vi "init.vi"(10 "Size":u32, 11 "Key Value Pairs":T1[](array[typedef])) -> (0 "error out":errorcluster, 3 "Bucket out":refnum<class "Bucket.lvclass">)   [LabVIEW 2017, in "Bucket.lvclass"]
uses:
  <userlib>/836-Library/Data_Structures/Bucket/Bucket.lvclass
  <userlib>/836-Library/Data_Structures/Bucket/Types/KeyValuePair.ctl
  <userlib>/836-Library/Data_Structures/Bucket/Bucket.lvclass/Bucket.ctl
  <vilib>/Utility/error.llb/Error Cluster From Error Code.vi
  <vilib>/ErrorRing/Error Ring.xnode
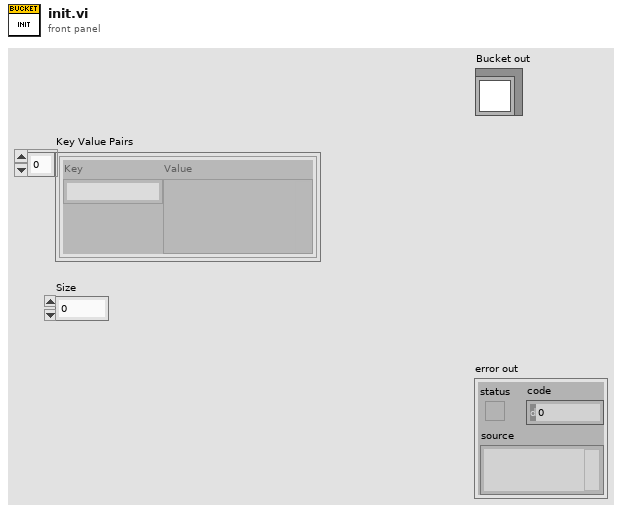
[diagram p1: front panel]
types:
  T1 = typedef "KeyValuePair.ctl" = cluster{"Key":string, "Value":variant}
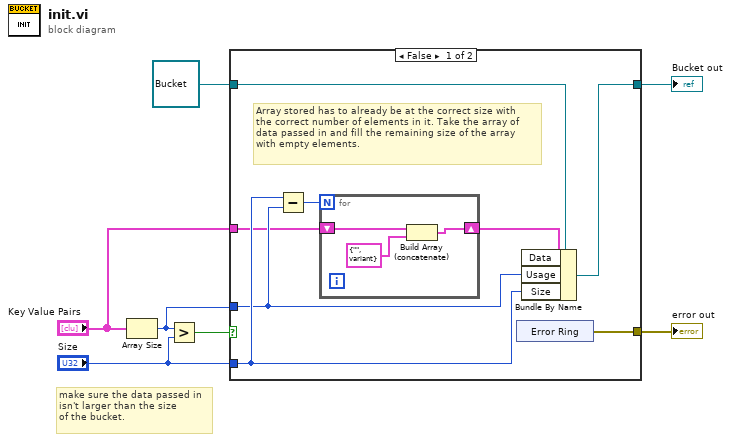
[diagram p0: block diagram]
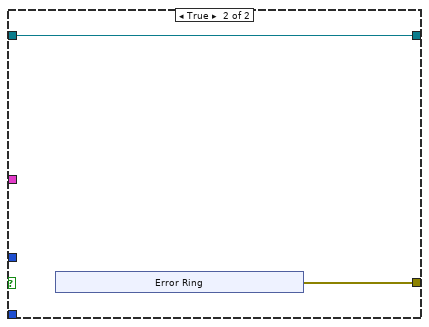
[diagram p2: hidden frame]
diagram:
  # "make sure the data passed in\nisn't larger than the size\nof the bucket."
  n1 = Array Size(array="Key Value Pairs") -> (size(s)=w1:i32)
  n2 = Greater?(x=w1, y="Size") -> (0:w4:bool)
  n3 = case shown="False" w4 {
    tunnel: refnum<class "Bucket.lvclass"> refnum ("Bucket in") -> [w15 w21]
    tunnel: [w13 w21] -> w5
    tunnel: [w14 w20] -> w7
    tunnel: "Key Value Pairs" -> [w9 _]
    tunnel: "Size" -> [w12 _]
    tunnel: w1 -> [w11 _]
    frame False {
      # "Array stored has to already be at the correct size with\nthe correct number of elements in it. Take the array of\ndata passed in and fill the remaining size of the array\nwith empty elements."
      n4 = Subtract(x=w12, y=w11) -> (x-y=w10:u32)
      n5 = for {
        N: w10 -> [_]
        shift-right: [w16] -> w8
        shift-left: w9 -> [w18]
        n6 = Build Array (concatenate)(w18, T1 {"Key"="", "Value"=variant} ("Cluster")) -> (w16:T1[])
      }
      n7 = xnode "Error Ring"() -> ("error out"=w14:errorcluster)
      n8 = Bundle By Name(cluster=w15, "Data"=w8, "Usage"=w11, "Size"=w12) -> (w13:refnum<class "Bucket.lvclass">)
    }
    frame True {
      n9 = xnode "Error Ring"() -> ("error out"=w20:errorcluster)
    }
  }
  "error out" <- w7
  "Bucket out" <- w5
